vi "MCL Read Encoder Z.vi"(8 "error in (no error)":errorcluster, 11 "handle":i32) -> (0 "error out":errorcluster, 3 "function return":dbl)   [LabVIEW 2014, in "Madlib.lvlib"]
doc: "MADLIB_API double MCL_ReadEncoderZ(int handle);"
uses:
  <userlib>/Lambda2/lib/Madlib/Madlib.lvlib
  <userlib>/Lambda2/lib/Madlib/Madlib.dll
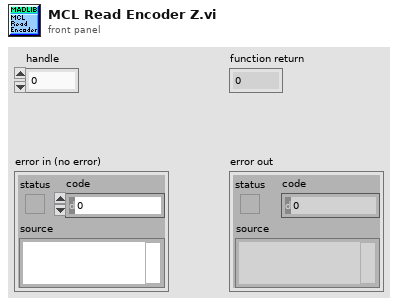
[diagram p1: front panel]
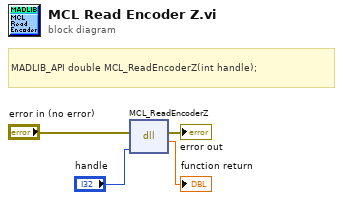
[diagram p0: block diagram]
diagram:
  # "MADLIB_API\tdouble\tMCL_ReadEncoderZ(int handle);"
  n1 = dll-call lib="C:/Program Files (x86)/National Instruments/LabVIEW 2014/user.lib/Lambda2/lib/Madlib/Madlib.*" fn="MCL_ReadEncoderZ"(error in="error in (no error)", "handle"="handle") -> (error out=→"error out":errorcluster, →"function return":dbl)  [unwired: 3 in, 1 out]
